vi "Word Open method.vi"(0 "Word.Documents":refnum<k7>, 7 "FileName":path, 11 "error in (no error)":errorcluster) -> (4 "Open":refnum<k7>, 15 "error out":errorcluster)   [LabVIEW 2010]
panel:
  # "This VI is saved in LabVIEW 8.5 so that the  Word.Documents Open method will get mutated by LabVIEW to match the installed Office package."
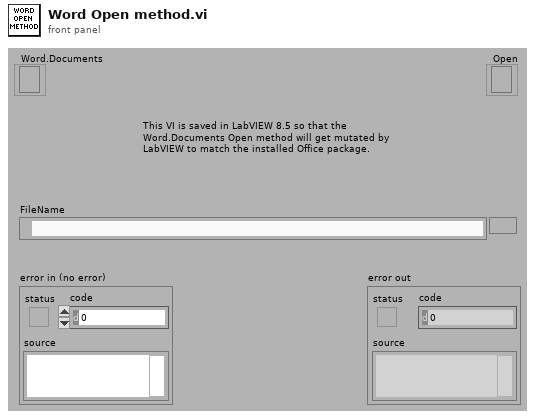
[diagram p1: front panel]
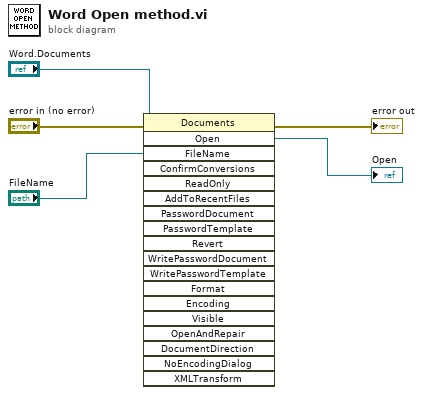
[diagram p0: block diagram]
diagram:
  n1 = invoke class="Documents" method="Open"(reference="Word.Documents", error in="error in (no error)", "FileName"="FileName") -> (error out=→"error out":errorcluster, "Open"=→"Open":refnum<k7>)  [unwired: 16 in, 17 out]
